vi "Meas Close Samples Stream MAT Variable.vi"(7 "Close MAT file? (False)":bool, 8 "error in":errorcluster, 11 "stream session":T1) -> (0 "error out":errorcluster, 2 "written samples":i64, 3 "MAT file ref out":refnum<file>)   [LabVIEW 2020]
doc: "Closes streamed variable in the MAT file. It will update preallocated size of the file and variable header according to the actually written data. Optionally it can also close the whole MAT file. Otherwise it will return valid reference to the opened MAT file for further use."
uses:
  Meas Samples Stream.ctl
  octave/mat/MAT Type Representation.ctl
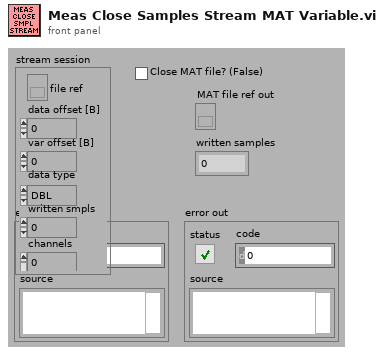
[diagram p1: front panel]
types:
  T1 = typedef "Meas Samples Stream.ctl" = cluster{"file ref":refnum<file>, "data offset [B]":i64, "var offset [B]":i64, "data type":T2, "written smpls":i64, "channels":i64}
  T2 = typedef "MAT Type Representation.ctl" = enum16{"DBL", "SGL", "I32", "I16", "U16", "U8", "CDB", "CSG", "STR"}
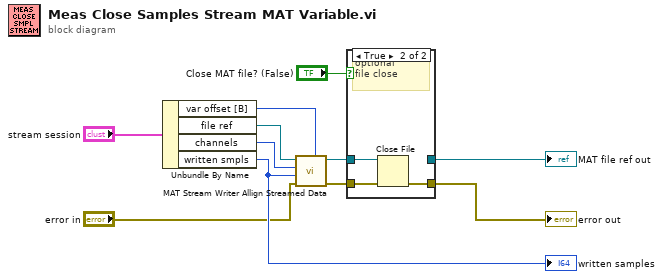
[diagram p0: block diagram]
diagram:
  n1 = Unbundle By Name("stream session") -> ("var offset [B]"=w9:i64, "file ref"=w10:refnum<file>, "channels"=w8:i64, "written smpls"=w7:i64)
  "written samples" <- w7
  n2 = call "MAT Stream Writer Allign Streamed Data.vi"("variable header offset (0: file start)"=w9, "error in (no error)"="error in", "columns count"=w7, "rows count"=w8, "Ref Num"=w10) -> ("error out"=w6:errorcluster, "Dup Ref Num"=w5:refnum<file>)  [unwired: 4 in, 1 out]
  n3 = case shown="True" "Close MAT file? (False)" {
    tunnel: w6 -> [w13 w16]
    tunnel: w5 -> [w12 w15]
    tunnel: [w13 w14] -> w2
    tunnel: [w12 _] -> w3
    frame False {
    }
    frame True {
      # "optional\nfile close"
      n4 = Close File(refnum=w15, error in=w16) -> (error out=w14:errorcluster)  [unwired: 1 out]
    }
  }
  "error out" <- w2
  "MAT file ref out" <- w3
